vi "Set All Elements.vi"(8 "error in":errorcluster, 10 "Section Node":refnum<k20>, 11 "Section Ref in":refnum<data-value>) -> (0 "error out":errorcluster, 3 "Section Ref out":refnum<data-value>)   [LabVIEW 2024, in "Config File Parser.lvlib" / "Section.lvclass"]
uses:
  Section.lvclass
  <vilib>/xml/Close Reference(Node).vi
  Section.lvclass/Section.ctl
  <resource>/objmgr/DOMUserDefRef.rc
  Config File Parser.lvlib
  <vilib>/xml/NI_XML.lvlib
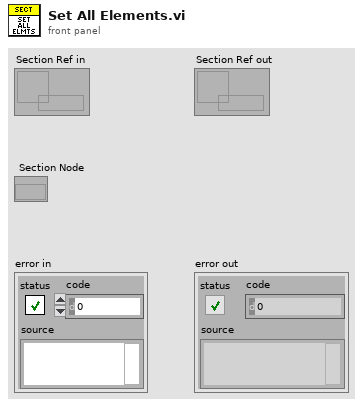
[diagram p1: front panel]
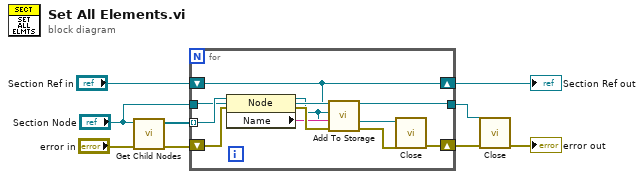
[diagram p0: block diagram]
diagram:
  n1 = call "Get Child Nodes.vi"("error in"="error in", "Node"="Section Node") -> ("error out"=w8:errorcluster, "Child Nodes"=w5:refnum<k20>[])  [unwired: 8 in]
  n2 = for {
    tunnel: w5 -> [w14] mode=indexing
    shift-right: [w15] -> w6
    shift-left: w8 -> [w18]
    tunnel: [w12] -> w3
    tunnel: "Section Node" -> [w12]
    shift-right: [w11] -> w1
    shift-left: "Section Ref in" -> [w11]
    n3 = property on="Property Node" class="Node"(reference=w14, error in=w18) -> (reference out=w10:refnum<k20>, error out=w17:errorcluster, "Name"=w13:string)
    n4 = call "Add To Storage.vi"("error in"=w17, "Item Name"=w13, "Item node"=w10, "Item Ref in"=w11) -> ("error out"=w16:errorcluster)  [unwired: 6 in, 1 out]
    n5 = call-poly <vilib>:"Close.vi"("error in (no error)"=w16, "node"=w10) -> ("error out"=w15:errorcluster)  [unwired: 7 in]
  }
  "Section Ref out" <- w1
  n6 = call-poly <vilib>:"Close.vi"("error in (no error)"=w6, "node"=w3) -> ("error out"=→"error out":errorcluster)  [unwired: 7 in]
